vi "Save Buffered Data.vi"(8 "error in (no error)":errorcluster, 11 "Interface Message Specifier in":refnum<class "Interface Message Specifier.lvclass">) -> (0 "error out":errorcluster, 3 "Interface Message Specifier out":refnum<class "Interface Message Specifier.lvclass">)   [LabVIEW 2020, in "Interface Message Specifier.lvlib" / "Interface Message Specifier.lvclass"]
uses:
  Interface Message Specifier.lvclass
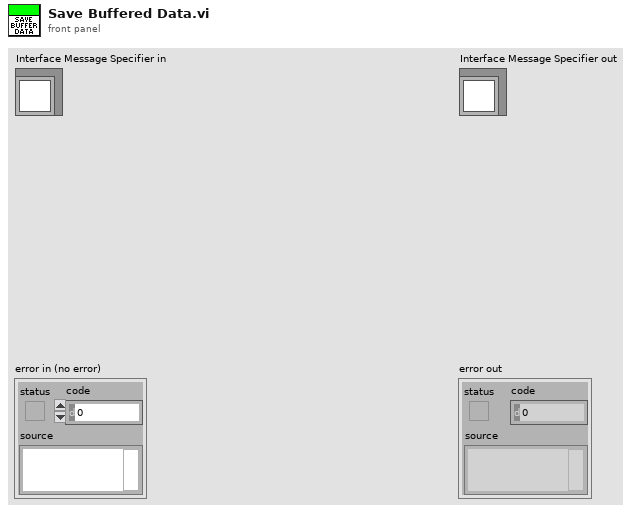
[diagram p1: front panel]
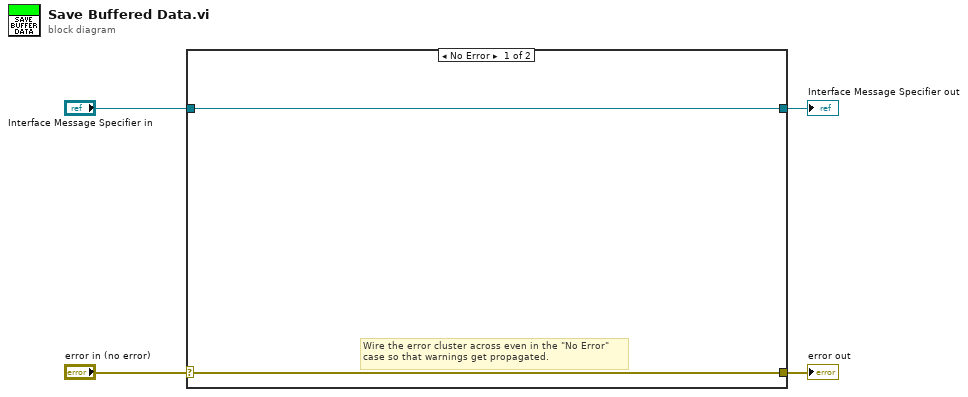
[diagram p0: block diagram]
diagram:
  n1 = case shown="No Error" "error in (no error)" {
    selector: "error in (no error)" -> [w5 w8]
    tunnel: [w5 w8] -> w3
    tunnel: [w6 w7] -> w1
    tunnel: "Interface Message Specifier in" -> [w6 w7]
    frame No Error {
      # "Wire the error cluster across even in the \"No Error\"\ncase so that warnings get propagated."
    }
    frame Error {
    }
  }
  "error out" <- w3
  "Interface Message Specifier out" <- w1
